vi "Find Bots from Scores.vi"(9 "Circle Scores":sgl[](array[numeric]), 10 "Square Scores":sgl[](array[numeric]), 11 "Bots":T1(array[cluster])) -> (1 "Triangle":T2, 2 "Circle":T2, 3 "Square":T2)   [LabVIEW 2018]
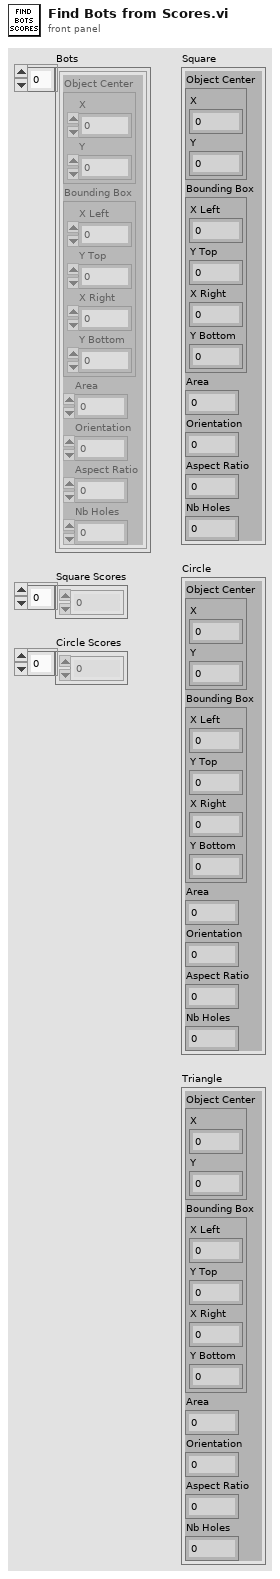
[diagram p1: front panel]
types:
  T1 = cluster{"Object Center":cluster{"X":sgl, "Y":sgl}, "Bounding Box":cluster{"X Left":i32, "Y Top":i32, "X Right":i32, "Y Bottom":i32}, "Area":sgl, "Orientation":sgl, "Aspect Ratio":sgl, "Nb Holes":i32}[]
  T2 = cluster{"Object Center":cluster{"X":sgl, "Y":sgl}, "Bounding Box":cluster{"X Left":i32, "Y Top":i32, "X Right":i32, "Y Bottom":i32}, "Area":sgl, "Orientation":sgl, "Aspect Ratio":sgl, "Nb Holes":i32}
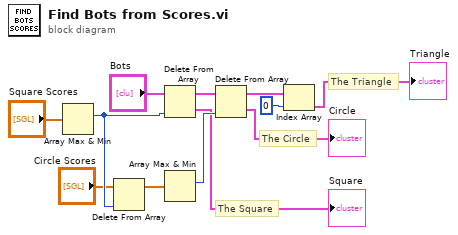
[diagram p0: block diagram]
diagram:
  # "The Triangle"
  # "The Circle"
  # "The Square"
  n1 = Array Max & Min(array="Square Scores") -> (max index (indices)=w3:i32)  [unwired: 3 out]
  n2 = Delete From Array(array="Circle Scores", index=w3) -> (array with subset deleted=w6:sgl[])  [unwired: 1 in, 1 out]
  n3 = Delete From Array(array="Bots", index=w3) -> (deleted portion=→"Square":T2, array with subset deleted=w8:T1)  [unwired: 1 in]
  n4 = Array Max & Min(array=w6) -> (max index (indices)=w7:i32)  [unwired: 3 out]
  n5 = Delete From Array(array=w8, index=w7) -> (deleted portion=→"Circle":T2, array with subset deleted=w10:T1)  [unwired: 1 in]
  n6 = Index Array(array=w10, index=0) -> (element=→"Triangle":T2)
